vi "PH_Beckhoff_PP_PU.set i Attr and start DIM Services for Ignitron.vi"(3 "error in":errorcluster, 4 "Values":T4, 5 "PU Type":T1=enum."PA 19mm") -> (0 "error out":errorcluster, 1 "Igni":T3(array[cluster]) {"Status"."Status" items=["no info", "off/false/out", "on/true/in", "Failure", "Alarm", "Status 1", "Status 2", "Status 3"]})   [LabVIEW 2014, in "PH_Beckhoff_PP_PU.lvlib"]
uses:
  PH_Beckhoff_PP_PU.lvlib
  PH_Beckhoff/PH_Beckhoff.Values.ctl
  PH_Beckhoff/PH_Beckhoff.Sonderklemmen Inputs.ctl
  PH_Beckhoff/PH_Beckhoff.Analog Inputs.ctl
  PH_Beckhoff/PH_Beckhoff.Scaling Type.ctl
  PH_Beckhoff/PH_Beckhoff.Analog Outputs.ctl
  PH_Beckhoff/PH_Beckhoff.Digital Inputs.ctl
  PH_Beckhoff/PH_Beckhoff.Digital Outputs.ctl
  PH_Basics/PH_StatusHandler/PH_StatusHandler.Status.ctl
  PH_Beckhoff_PP_PU.PU Rack Type.ctl
  PH_Beckhoff_PP_PU.Igni Tags.ctl
  PH_Basics/PH_PP_Common/PH_PP_Common.PUs.ctl
  CSlibraries-extern/DimLVEvent/LVDimInterface/LVDimInterface.lvlib
  PH_Basics/PH_StatusHandler/PH_StatusHandler.lvlib
  PH_Basics/PH_PP_Common/PH_PP_Common.lvlib
  PH_Beckhoff/PH_Beckhoff.lvlib
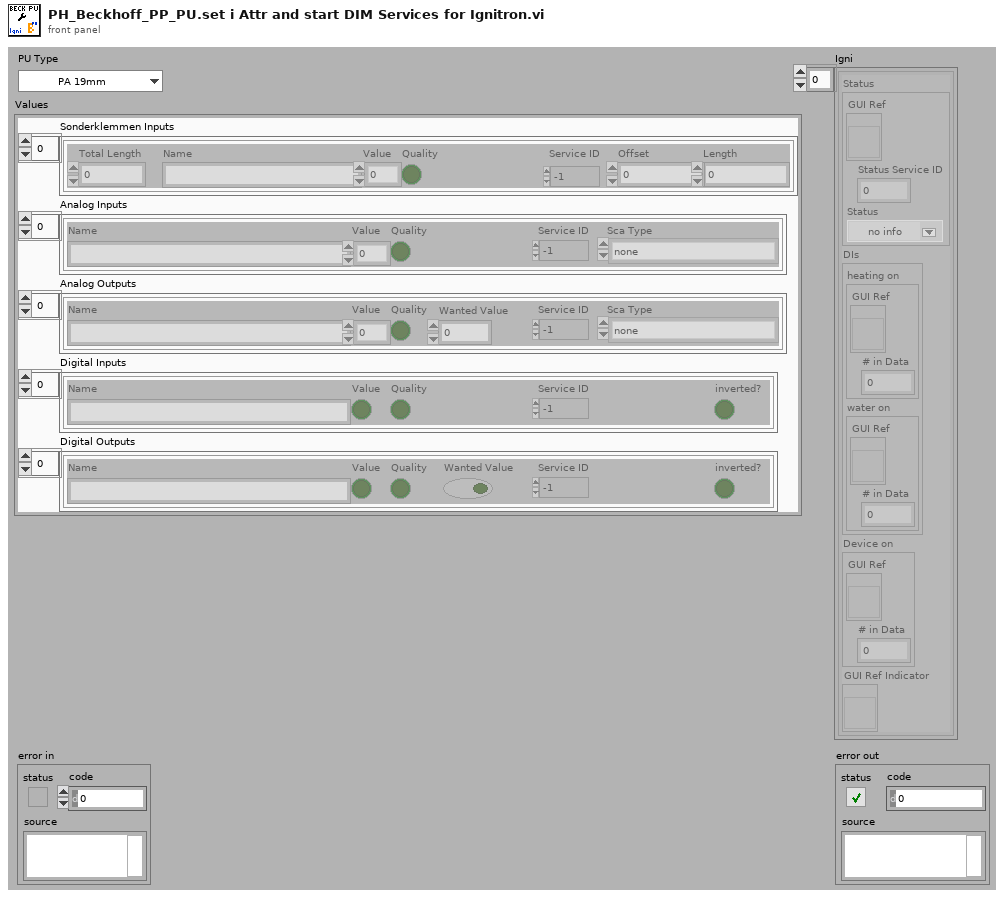
[diagram p1: front panel]
types:
  T1 = typedef "PH_Beckhoff_PP_PU.lvlib/PH_Beckhoff_PP_PU.PU Rack Type.ctl" = enum16{"no Info", "PA 19mm", "PA 45mm", "MA PU 1 and 2", "MA PU 3 and 4", "MA PU 5 and 6", "MA FR and PILC"}
  T2 = typedef "PH_StatusHandler.lvlib/PH_StatusHandler.Status.ctl" = i16
  T3 = cluster{"Status":cluster{"GUI Ref":refnum<vi>, "Status Service ID":i32, "Status":T2}, "DIs":cluster{"heating on":cluster{"GUI Ref":refnum<vi>, "# in Data":i32}, "water on":cluster{"GUI Ref":refnum<vi>, "# in Data":i32}}, "Device on":cluster{"GUI Ref":refnum<vi>, "# in Data":i32}, "GUI Ref Indicator":refnum<vi>}[]
  T4 = typedef "PH_Beckhoff.lvlib/PH_Beckhoff.Values.ctl" = cluster{"Sonderklemmen Inputs":T5, "Analog Inputs":T6, "Analog Outputs":T8, "Digital Inputs":T9, "Digital Outputs":T10}
  T5 = typedef "PH_Beckhoff.lvlib/PH_Beckhoff.Sonderklemmen Inputs.ctl" = cluster{"Total Length":u32, "Name":string, "Value":u64, "Quality":bool, "Service ID":i32, "Offset":u32, "Length":u32}[]
  T6 = typedef "PH_Beckhoff.lvlib/PH_Beckhoff.Analog Inputs.ctl" = cluster{"Name":string, "Value":u32, "Quality":bool, "Service ID":i32, "Sca Type":T7}[]
  T7 = typedef "PH_Beckhoff.lvlib/PH_Beckhoff.Scaling Type.ctl" = enum16{"none", "0 ... 15 Bit -> 0 ... 5", "0 ... 15 Bit -> 0 ... 10", "0 ... 15 Bit -> 0 ... 25", "0 ... 15 Bit -> 4 ... 20", "0 ... 15 Bit -> 0 ... 1", "0 ... 15 Bit -> 0 ... 20000", "0 ... 15 Bit -> 0 ... 24000"}
  T8 = typedef "PH_Beckhoff.lvlib/PH_Beckhoff.Analog Outputs.ctl" = cluster{"Name":string, "Value":u32, "Quality":bool, "Wanted Value":u32, "Service ID":i32, "Sca Type":T7}[]
  T9 = typedef "PH_Beckhoff.lvlib/PH_Beckhoff.Digital Inputs.ctl" = cluster{"Name":string, "Value":bool, "Quality":bool, "Service ID":i32, "inverted?":bool}[]
  T10 = typedef "PH_Beckhoff.lvlib/PH_Beckhoff.Digital Outputs.ctl" = cluster{"Name":string, "Value":bool, "Quality":bool, "Wanted Value":bool, "Service ID":i32, "inverted?":bool}[]
  T11 = typedef "PH_Beckhoff_PP_PU.lvlib/PH_Beckhoff_PP_PU.Igni Tags.ctl" = enum16{"heating-on", "water-on", "Device-on", "Status"}
  T12 = typedef "PH_PP_Common.lvlib/PH_PP_Common.PUs.ctl" = enum16{"no Info", "PA-19mm-1", "PA-19mm-2", "PA-45mm-PILC", "PA-45mm-MAIN", "MA-PU-1", "MA-PU-2", "MA-PU-3", "MA-PU-4", "MA-PU-5", "MA-PU-6", "MA-FR", "MA-PILC", "PA-45mm-DP"}
  T13 = cluster{"Status":cluster{"GUI Ref":refnum<vi>, "Status Service ID":i32, "Status":T2}, "DIs":cluster{"heating on":cluster{"GUI Ref":refnum<vi>, "# in Data":i32}, "water on":cluster{"GUI Ref":refnum<vi>, "# in Data":i32}}, "Device on":cluster{"GUI Ref":refnum<vi>, "# in Data":i32}, "GUI Ref Indicator":refnum<vi>}
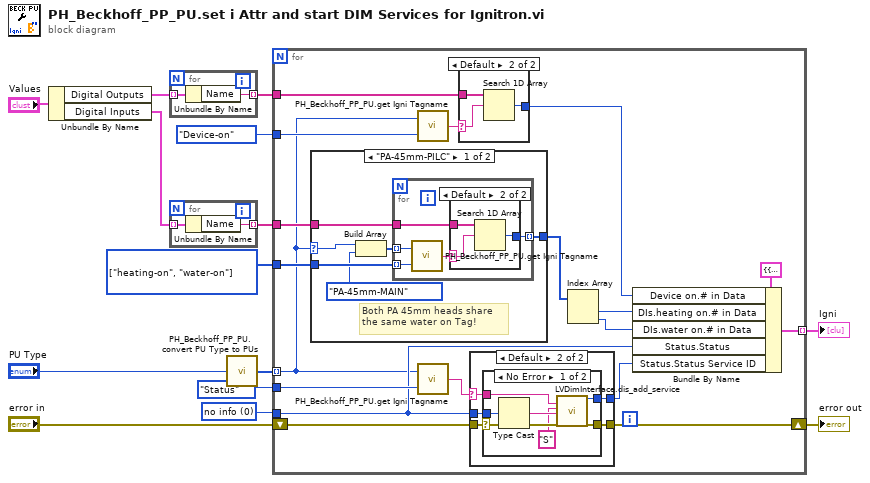
[diagram p0: block diagram]
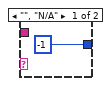
[diagram p2: hidden frame]
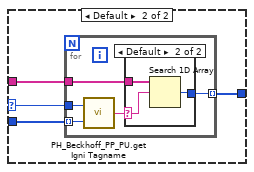
[diagram p3: hidden frame]
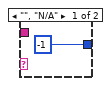
[diagram p4: hidden frame]
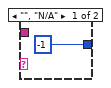
[diagram p5: hidden frame]
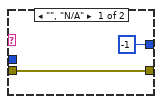
[diagram p6: hidden frame]
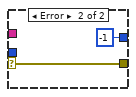
[diagram p7: hidden frame]
diagram:
  w5 = T11[] [enum."heating-on", enum."water-on"] items=["heating-on", "water-on", "Device-on", "Status"]
  w11 = T2 0 items=["no info", "off/false/out", "on/true/in", "Failure", "Alarm", "Status 1", "Status 2", "Status 3"] ("Status")
  n1 = Unbundle By Name("Values") -> ("Digital Outputs"=w9:T10, "Digital Inputs"=w7:T9)
  n2 = for {
    tunnel: w9 -> [w16] mode=indexing
    tunnel: [w15] -> w8 mode=indexing
    n3 = Unbundle By Name(w16) -> ("Name"=w15:string)
  }
  n4 = for {
    tunnel: w7 -> [w18] mode=indexing
    tunnel: [w17] -> w6 mode=indexing
    n5 = Unbundle By Name(w18) -> ("Name"=w17:string)
  }
  n6 = call "PH_Beckhoff_PP_PU.convert PU Type to PUs.vi"("PU Type"="PU Type") -> ("PUs"=w13:T12[])
  n7 = for {
    shift-right: [w33] -> w4
    shift-left: "error in" -> [w34]
    tunnel: [w36] -> w1 mode=indexing
    tunnel: w13 -> [w20] mode=indexing
    tunnel: PH_Beckhoff_PP_PU.Igni_Tags."Status" ("Igni Tag") -> [w35]
    tunnel: w11 -> [w30]
    tunnel: PH_Beckhoff_PP_PU.Igni_Tags."Device-on" ("Igni Tag") -> [w29]
    tunnel: w8 -> [w27]
    tunnel: w6 -> [w25]
    tunnel: w5 -> [w24]
    n8 = case shown="\"PA-45mm-PILC\"" w20 {
      selector: w20 -> [w39 w52]
      tunnel: w25 -> [w42 w55]
      tunnel: w24 -> [w41 w54]
      tunnel: [w40 w53] -> w23
      frame "PA-45mm-PILC" {
        # "Both PA 45mm heads share\nthe same water on Tag!"
        n9 = Build Array(w39, PH_PP_Common.PUs."PA-45mm-MAIN" ("element")) -> (w38:T12[])
        n10 = for {
          tunnel: w38 -> [w47] mode=indexing
          tunnel: w42 -> [w46]
          tunnel: w41 -> [w45] mode=indexing
          tunnel: [w44] -> w40 mode=indexing
          n11 = call "PH_Beckhoff_PP_PU.get Igni Tagname.vi"("Igni Tag"=w45, "PU"=w47) -> ("Igni Tagname"=w43:string)
          n12 = case shown="Default" w43 {
            selector: w43 -> [_ w51]
            tunnel: [-1 ("my_serviceID") w49] -> w44
            tunnel: w46 -> [_ w50]
            frame "", "N/A" {
            }
            frame Default {
              n13 = Search 1D Array(1D array=w50, element=w51) -> (index of element=w49:i32)  [unwired: 1 in]
            }
          }
        }
      }
      frame Default {
        n14 = for {
          tunnel: w52 -> [w60]
          tunnel: w55 -> [w59]
          tunnel: w54 -> [w58] mode=indexing
          tunnel: [w57] -> w53 mode=indexing
          n15 = call "PH_Beckhoff_PP_PU.get Igni Tagname.vi"("Igni Tag"=w58, "PU"=w60) -> ("Igni Tagname"=w56:string)
          n16 = case shown="Default" w56 {
            selector: w56 -> [_ w64]
            tunnel: [-1 ("my_serviceID") w62] -> w57
            tunnel: w59 -> [_ w63]
            frame "", "N/A" {
            }
            frame Default {
              n17 = Search 1D Array(1D array=w63, element=w64) -> (index of element=w62:i32)  [unwired: 1 in]
            }
          }
        }
      }
    }
    n18 = call "PH_Beckhoff_PP_PU.get Igni Tagname.vi"("Igni Tag"=w29, "PU"=w20) -> ("Igni Tagname"=w28:string)
    n19 = call "PH_Beckhoff_PP_PU.get Igni Tagname.vi"("Igni Tag"=w35, "PU"=w20) -> ("Igni Tagname"=w32:string)
    n20 = case shown="Default" w28 {
      selector: w28 -> [_ w68]
      tunnel: [-1 ("my_serviceID") w66] -> w26
      tunnel: w27 -> [_ w67]
      frame "", "N/A" {
      }
      frame Default {
        n21 = Search 1D Array(1D array=w67, element=w68) -> (index of element=w66:i32)  [unwired: 1 in]
      }
    }
    n22 = case shown="Default" w32 {
      selector: w32 -> [_ w71]
      tunnel: w34 -> [w70 w75]
      tunnel: [w70 w74] -> w33
      tunnel: [-1 ("my_serviceID") w73] -> w31
      tunnel: w30 -> [_ w72]
      frame "", "N/A" {
      }
      frame Default {
        n23 = case shown="No Error" w75 {
          selector: w75 -> [w80 w84]
          tunnel: [w82 -1 ("my_serviceID")] -> w73
          tunnel: [w81 w84] -> w74
          tunnel: w72 -> [w79 _]
          tunnel: w71 -> [w76 _]
          frame No Error {
            n24 = Type Cast(x=w79) -> (*(type *) &x=w78:string)  [unwired: 1 in]
            n25 = call "LVDimInterface.dis_add_service.vi"("serviceName"=w76, "typeDescriptor"="S", "data"=w78, "error in (no error)"=w80) -> ("my_serviceID"=w82:i32, "error out"=w81:errorcluster)  [unwired: 14 in]
          }
          frame Error {
          }
        }
      }
    }
    n26 = Index Array(array=w23) -> (element #1=w22:i32, element #2=w21:i32)  [unwired: 2 in]
    n27 = Bundle By Name(cluster=T13 {"Status"={"GUI Ref"=refnum, "Status Service ID"=0, "Status"=0}, "DIs"={"heating on"={"GUI Ref"=refnum, "# in Data"=0}, "water on"={"GUI Ref"=refnum, "# in Data"=0}}, "Device on"={"GUI Ref"=refnum, "# in Data"=0}, "GUI Ref Indicator"=refnum} ("Igni Data"), "Device on.# in Data"=w26, "DIs.heating on.# in Data"=w22, "DIs.water on.# in Data"=w21, "Status.Status"=w30, "Status.Status Service ID"=w31) -> (w36:T13)
  }
  "Igni" <- w1
  "error out" <- w4
